vi "RC Decay acquisition loop.vi"(7 "Timing Control Parameters In":T1={"N cycles for averaging"=100, "N points per measurement"=1000, "Measurment time interval"=1e-05} {"Measurment time interval" format="%.2e"}, 11 "error in (no error)":errorcluster) -> (3 "time-out?":bool, 4 "data valid":bool=TRUE, 8 "Normalized Waveform Out":waveform(dbl)={"t0"=timestamp(3255113673.8489995 s since 1904-01-01), "dt"=9.999999747378752e-06, "Y"=array[1000 elements]}, 10 "Timing Control Parameters Out":T1={"N cycles for averaging"=300, "N points per measurement"=1000, "Measurment time interval"=1e-05} {"Measurment time interval" format="%.2e"}, 15 "error out":errorcluster)   [LabVIEW 2014]
doc: "This subvi manages the capacitance measurement\n\nPaul K Dixon\nPhysics 350\nCSUSB Physics"
uses:
  globals/C(T) global variables.vi
panel:
  out "data":waveform(dbl)[](array[waveform])=[{"t0"=timestamp(3255113673.8489995 s since 1904-01-01), "dt"=9.999999747378752e-06, "Y"=array[1000 elements], "attributes"=variant("NI_ChannelName"=variant(string "1"), "NI_DeviceNumber"=variant(i32 1), "NI_UnitDescription"=variant(string "Volts"))}, {"t0"=timestamp(3255113673.8489995 s since 1904-01-01), "dt"=9.999999747378752e-06, "Y"=array[1000 elements], "attributes"=variant("NI_ChannelName"=variant(string "2"), "NI_DeviceNumber"=variant(i32 1), "NI_UnitDescription"=variant(string "Volts"))}] caption="Individual Waveforms"
  out "Individual Waveforms":waveform(dbl)[](graph)
  out "Final Waveform":waveform(dbl)(graph)={"t0"=timestamp(3255113673.8489995 s since 1904-01-01), "dt"=9.999999747378752e-06, "Y"=[]}
  out "loop index":i32=300
  out "scan rate (Hz)":dbl=99999.99999999999 format="%.2e"
  out "meas index":i32=300
  in  "Proceed":bool
  # "RC Decay Acquisition for C(T) Experiment"
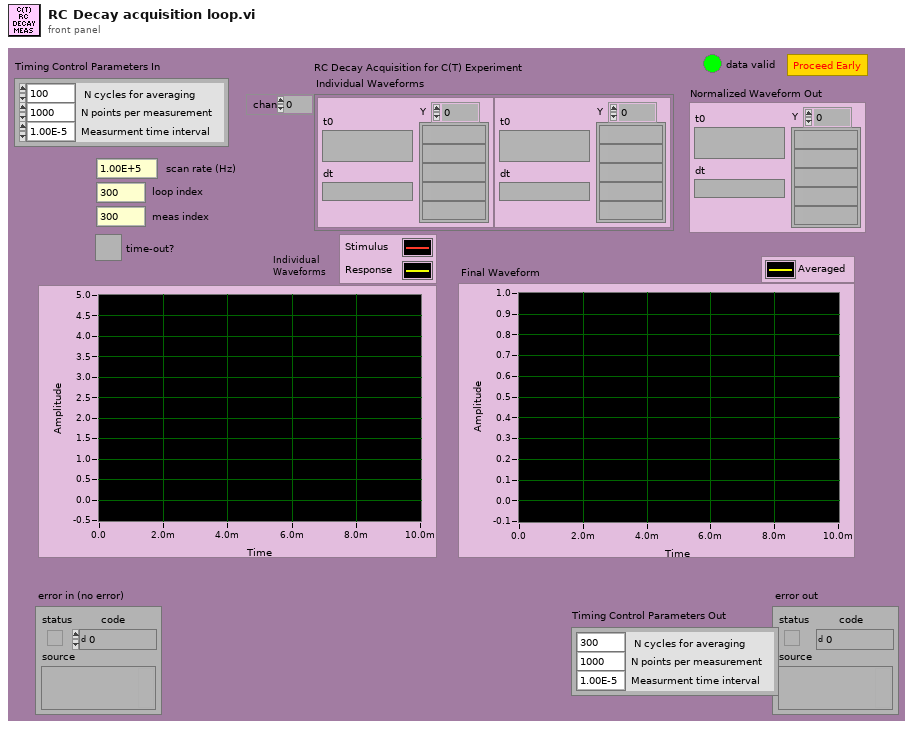
[diagram p1: front panel]
types:
  T1 = cluster{"N cycles for averaging":i32, "N points per measurement":i32, "Measurment time interval":dbl}
  T2 = enum16{"AI sample channel scan", "AI Waveform triggered"}
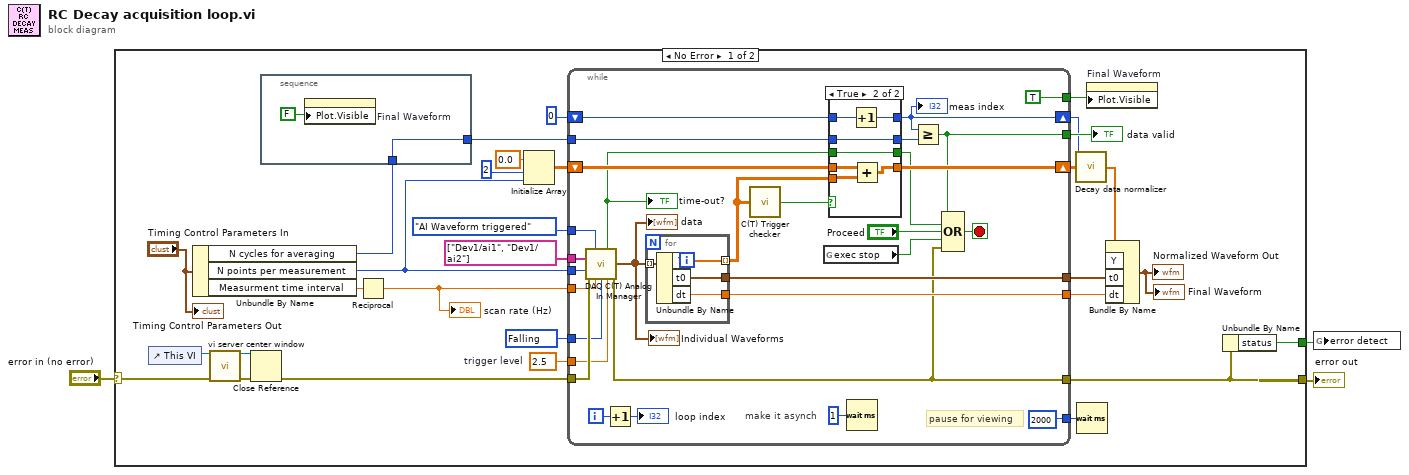
[diagram p0: block diagram]
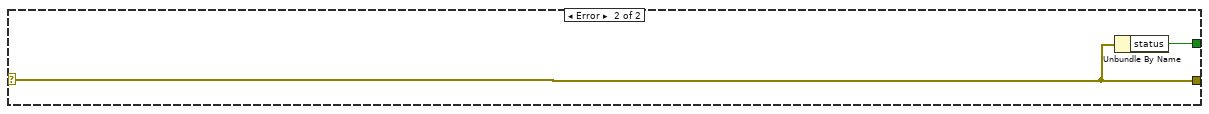
[diagram p3: hidden frame]
diagram:
  n1 = case shown="No Error" "error in (no error)" {
    selector: "error in (no error)" -> [w10 w82]
    tunnel: [w5 w82] -> w3
    tunnel: [w4 w81] -> w1
    frame No Error {
      w15 = 2.5  # trigger level
      w11 = 10171 items=["Rising"=10280, "Falling"=10171] ("trigger edge")
      n2 = control-ref of="This VI"() -> (w9:refnum<vi>)
      n3 = Unbundle By Name("Timing Control Parameters In") -> ("N cycles for averaging"=w18:i32, "N points per measurement"=w25:i32, "Measurment time interval"=w27:dbl)
      n4 = call "vi server center window.vi"("VI ref in"=w9, "error in"=w10) -> ("VI ref out"=w6:refnum<vi>, "error out"=w8:errorcluster)  [unwired: 12 out]
      n5 = Close Reference(reference=w6, error in (no error)=w8) -> (error out=w7:errorcluster)
      n6 = stacked-sequence {
        tunnel: [w79] -> w17
        tunnel: w18 -> [w79]
        frame #0 {
          n7 = property on="Final Waveform" class="WFGraph (strict)"("Plot.Visible"=FALSE) -> ()  [unwired: 2 in, 2 out]
        }
      }
      n8 = Reciprocal(x=w27) -> (1/x=w26:dbl)
      "scan rate (Hz)" <- w26
      n9 = Initialize Array(0.0 ("Element Data"), 2 ("Dimension Size"), w25) -> (w31:dbl[][])
      n10 = while {
        tunnel: [TRUE ("Plot.Visible")] -> w16
        tunnel: [w48] -> w19
        tunnel: [w49] -> w14
        tunnel: [w51] -> w24
        tunnel: w17 -> [w55]
        shift-left: 0 ("Dimension Size") -> [w58]
        shift-right: [w54] -> w22
        tunnel: w26 -> [w60]
        tunnel: T2."AI Waveform triggered" ("AI mode chooser") -> [w61]
        tunnel: w25 -> [w62]
        shift-left: w31 -> [w57]
        shift-right: [w56] -> w23
        tunnel: w15 -> [w43]
        tunnel: [u32 2000 ("milliseconds to wait")] -> w13
        tunnel: w7 -> [w63]
        tunnel: [w34] -> w5
        tunnel: tag[] ["Dev1/ai1", "Dev1/ai2"] ("Channels (Triggered Waveform)") -> [w36]
        tunnel: w11 -> [w35]
        i -> [w52]
        stop <- w40 stop-if-true
        # "pause for viewing"
        # "make it asynch"
        n11 = call "DAQ C(T) Analog In Manager.vi"("AI mode chooser"=w61, "Channels (Triggered Waveform)"=w36, "number of scans to acquire"=w62, "error in (no error)"=w63, "scan rate"=w60, "trigger edge"=w35, "trigger level"=w43) -> ("Timed Out"=w37:bool, "data"=w45:waveform(dbl)[], "error out"=w34:errorcluster)  [unwired: 4 in, 2 out]
        "time-out?" <- w37
        "Individual Waveforms" <- w45
        "data" <- w45
        n12 = Increment(x=w52) -> (x+1=→"loop index":i32)
        n13 = for {
          tunnel: w45 -> [w78] mode=indexing
          tunnel: [w75] -> w42 mode=indexing
          tunnel: [w76] -> w49
          tunnel: [w77] -> w48
          n14 = Unbundle By Name(w78) -> ("Y"=w75:dbl[], "t0"=w76:timestamp, "dt"=w77:dbl)
        }
        n15 = call "C(T) Trigger checker.vi"("Raw C(T) data array"=w42) -> ("trigger was correct polarity"=w59:bool)
        n16 = global read "C(T) global variables.vi" "exec stop"() -> (w39:bool)
        n17 = case shown="True" w59 {
          tunnel: w42 -> [_ w71]
          tunnel: w58 -> [w67 w74]
          tunnel: [w67 w73] -> w54
          tunnel: w57 -> [w66 w72]
          tunnel: [w66 w70] -> w56
          tunnel: [w65 w69] -> w53
          tunnel: w55 -> [w65 w69]
          tunnel: [w64 w68] -> w38
          tunnel: w37 -> [w64 w68]
          frame False {
          }
          frame True {
            n18 = Increment(x=w74) -> (x+1=w73:i32)
            n19 = Add(x=w72, y=w71) -> (x+y=w70:dbl[][])
          }
        }
        "meas index" <- w54
        n20 = Wait (ms)(milliseconds to wait=u32 1) -> ()  [unwired: 1 out]
        n21 = Greater Or Equal?(x=w54, y=w53) -> (x >= y?=w51:bool)
        n22 = Compound Arithmetic op=OR(w51, w38, "Proceed", w39, w34) -> (w40:bool)
      }
      "data valid" <- w24
      n23 = call "Decay data normalizer.vi"("Number of samples"=w22, "Raw summed data Array"=w23) -> ("Normalized Decay"=w20:dbl[])  [unwired: 13 out]
      n24 = Wait (ms)(milliseconds to wait=w13) -> ()  [unwired: 1 out]
      n25 = property on="Final Waveform" class="WFGraph (strict)"("Plot.Visible"=w16) -> ()  [unwired: 2 in, 2 out]
      n26 = Bundle By Name("Y"=w20, "t0"=w14, "dt"=w19) -> (→"Normalized Waveform Out" →"Final Waveform":waveform(dbl))  [unwired: 1 out]
      n27 = Unbundle By Name(w5) -> ("status"=w4:bool)
      "Timing Control Parameters Out" <- "Timing Control Parameters In"
    }
    frame Error {
      n28 = Unbundle By Name(w82) -> ("status"=w81:bool)
    }
  }
  "error out" <- w3
  n29 = global write "C(T) global variables.vi" "error detect"(w1) -> ()
